vi "Welcome UI.vi"() -> ()   [LabVIEW 2016]
uses:
  <vilib>/Utility/error.llb/DialogType.ctl
  Architecture/Queue Management/ARC_Queue Create_Single.vi
  Architecture/Queue Management/ARC_Queue Valid.vi
  Architecture/Queue Management/ARC_Queue Insert Element.vi
  Architecture/Queue Management/ARC_Queue Remove Element.vi
  Architecture/Queue Management/ARC_Queue Destroy_Single.vi
panel:
  out "Logo":picture
  out "Title":string
  out "version":string
  in  "Parameter":cluster{"Q-Local":string, "Variant":variant}
  out "Error Report":string
  out "Current State":string
  in  "Exit Program":bool
  # "/* -------- Notes for All Users -------- */\nRecommand : \n[1].Display Setting Resolution -> 1440x900\n[2].Read Arch Notes First.\n[3].Make A Call When You Are In Trouble.\n\nTeam Members:\nPansino Soft,Pansino SDMA\n\nCopyright@2013 Pansino.Beijing\n\nVersion Number: 2013"
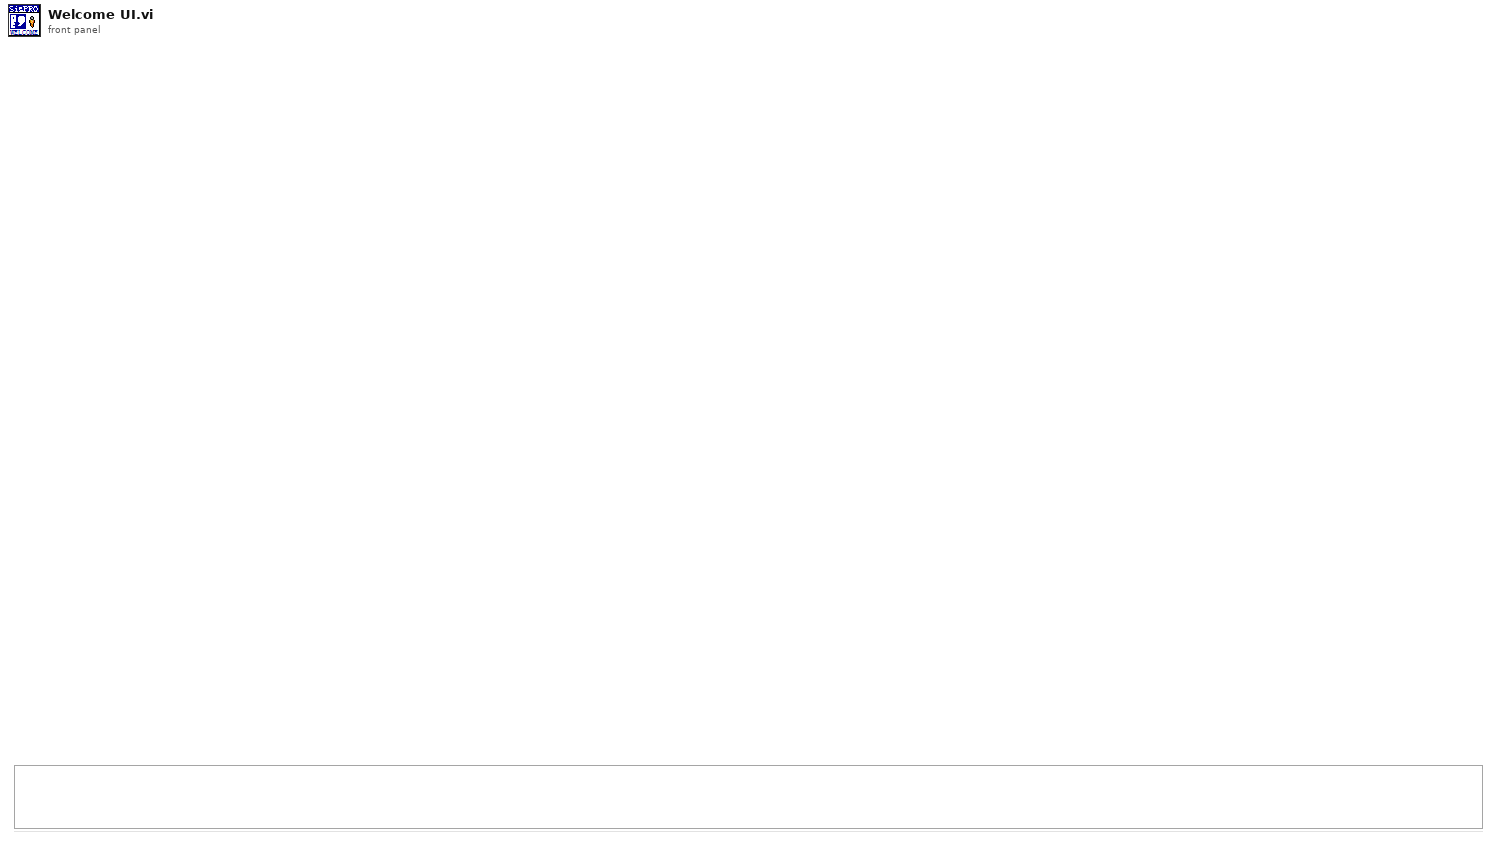
[diagram p1: front panel]
types:
  T1 = cluster{"Error":errorcluster, "Exit":bool, "System Path":cluster{"SysINI":path}, "Ref":cluster{"VIRef":refnum<vi>}, "Queue":cluster{"Q-Local":cluster{"Q-Local Name":string, "Q-Local Order":string, "Q-Local Data":variant}, "Q-HighLevel":cluster{"Q-HighLevel Name":string, "Q-HighLevel Order":string, "Q-HighLevel Data":variant}, "Q-LowLevel":cluster{"Q-LowLevel Name":string, "Q-LowLevel Order":string, "Q-LowLevel Data":variant}}}
  T2 = cluster{"LocalName":string, "System Config":path}
  T3 = typedef "DialogType.ctl" = u16
  T4 = cluster{"title":string, "version":string, "logo":path, "background":path}
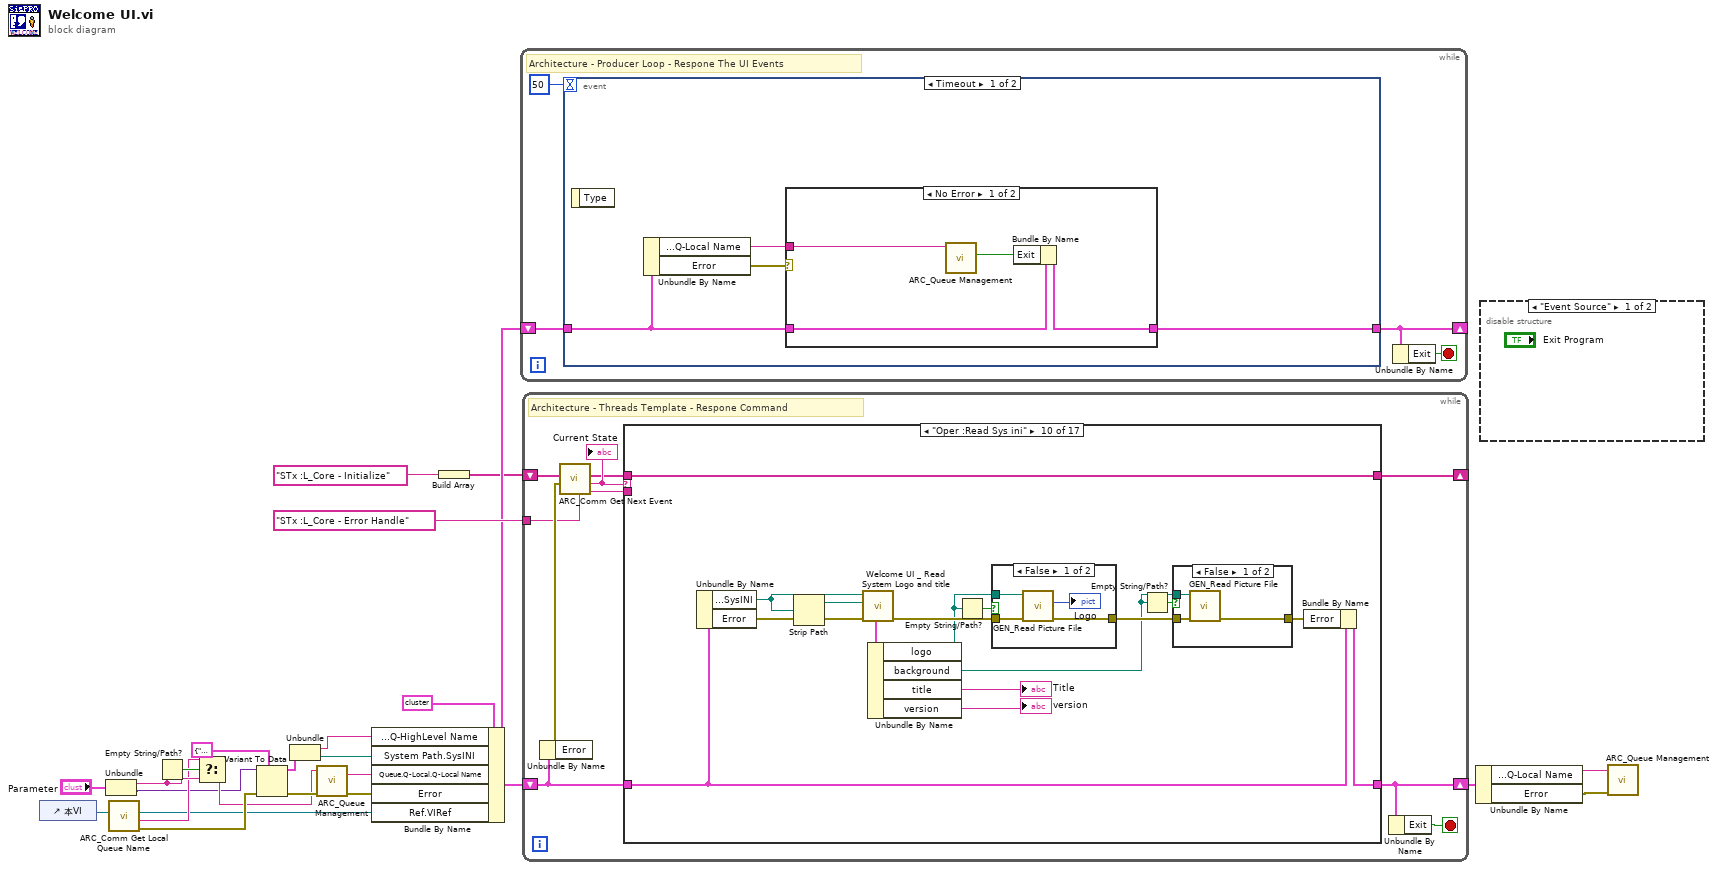
[diagram p0: block diagram]
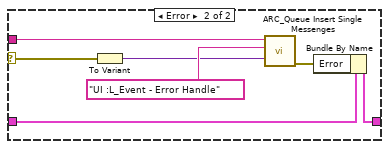
[diagram p2: hidden frame]
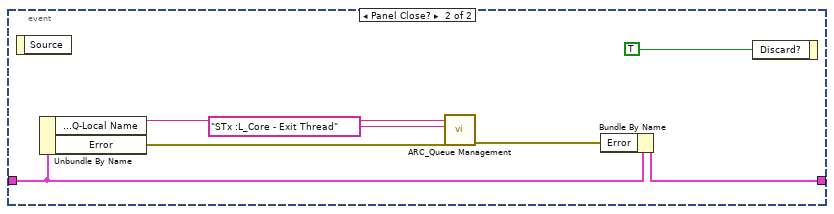
[diagram p3: hidden frame]
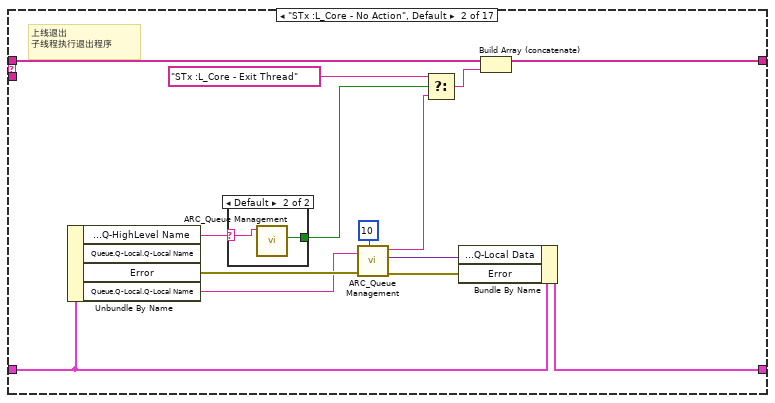
[diagram p6: hidden frame]
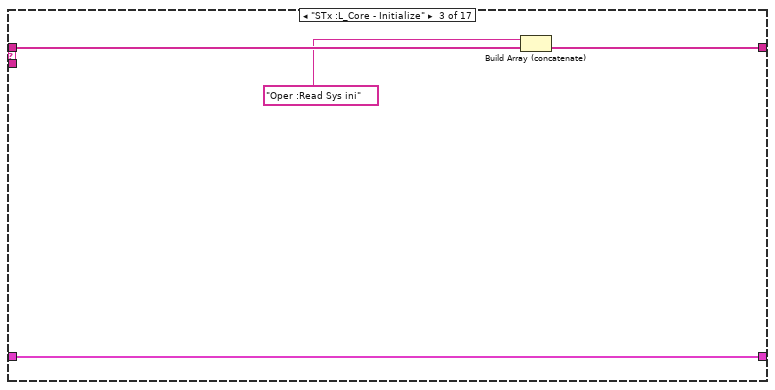
[diagram p8: hidden frame]
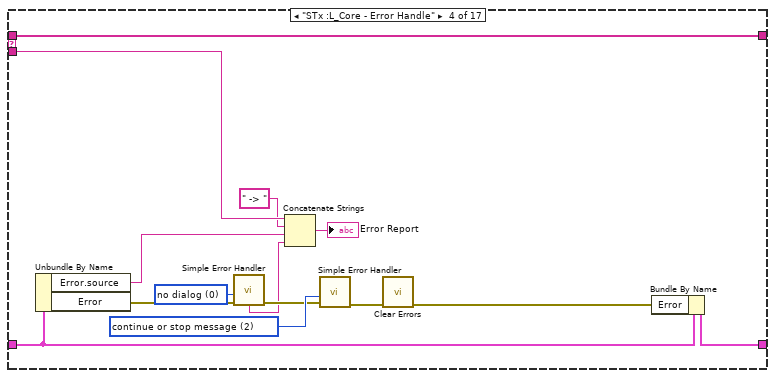
[diagram p9: hidden frame]
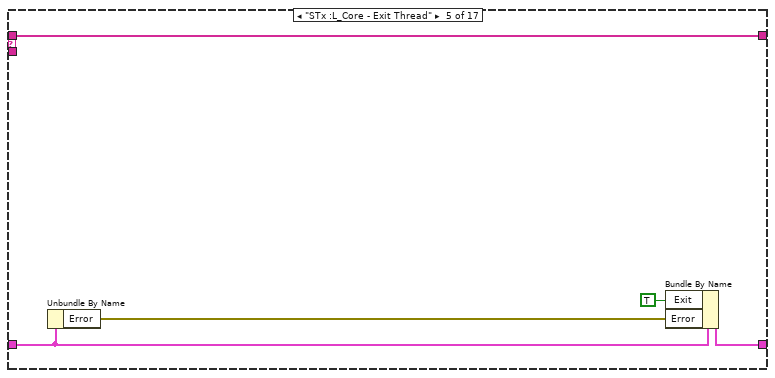
[diagram p10: hidden frame]
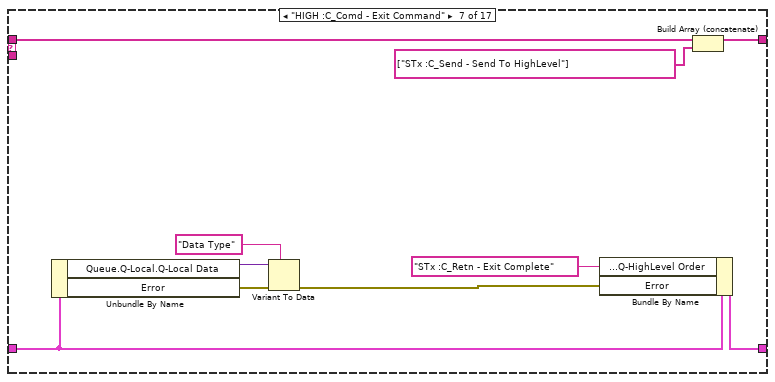
[diagram p12: hidden frame]
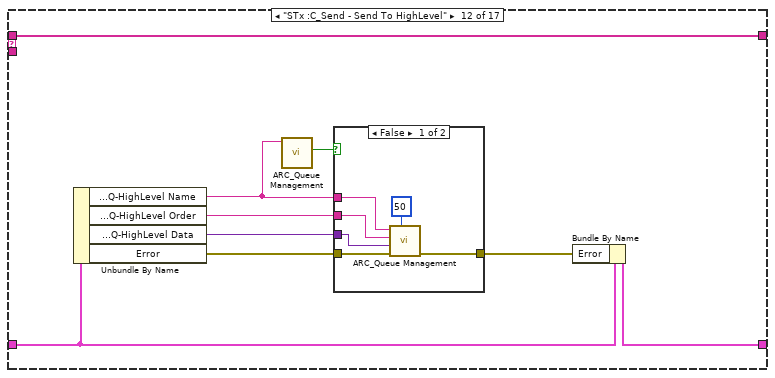
[diagram p18: hidden frame]
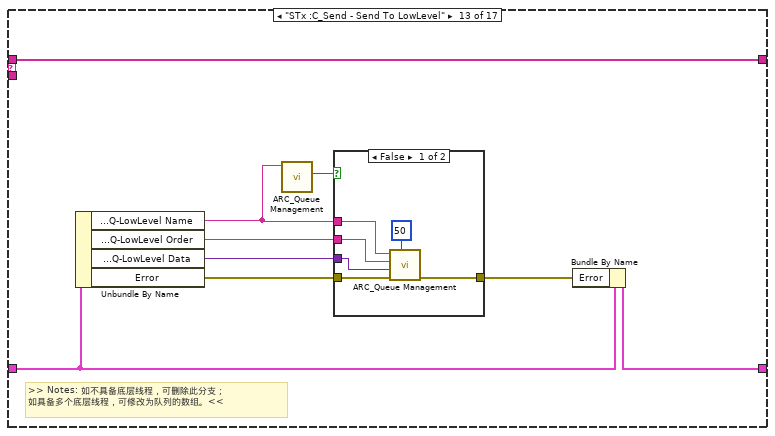
[diagram p20: hidden frame]
diagram:
  n1 = control-ref of="本VI"() -> (w13:refnum<vi>)
  n2 = Unbundle("Parameter") -> ("Q-Local"=w11:string, "Variant"=w6:variant)
  n3 = call "ARC_Comm Get Local Queue Name.vi"("VI Ref"=w13) -> ("error out"=w12:errorcluster, "VI  Name"=w9:string, "VI Ref out"=w5:refnum<vi>)  [unwired: 8 in]
  n4 = Empty String/Path?(string/path=w11) -> (empty?=w10:bool)
  n5 = Select(t=w9, s=w10, f=w11) -> (s? t:f=w8:string)
  n6 = Variant To Data(error in=w12, type=T2 {"LocalName"="", "System Config"=path ""} ("输出簇"), Variant=w6) -> (data=w3:T2, error out=w15:errorcluster)
  n7 = Unbundle(w3) -> ("LocalName"=w1:string, "System Config"=w2:path)
  n8 = call-poly "ARC_Queue Management.vi"("error in"=w15, "Queue Name"=w8) -> ("error out"=w24:errorcluster, "Queue Name dup"=w14:string)  [unwired: 7 in, 1 out]
  n9 = Bundle By Name(cluster=T1 {"Error"={"status"=FALSE, "code"=0, "source"=""}, "Exit"=FALSE, "System Path"={"SysINI"=path ""}, "Ref"={"VIRef"=refnum}, "Queue"={"Q-Local"={"Q-Local Name"="", "Q-Local Order"="", "Q-Local Data"=variant}, "Q-HighLevel"={"Q-HighLevel Name"="", "Q-HighLevel Order"="", "Q-HighLevel Data"=variant}, "Q-LowLevel"={"Q-LowLevel Name"="", "Q-LowLevel Order"="", "Q-LowLevel Data"=variant}}} ("TempVariable"), "Queue.Q-HighLevel.Q-HighLevel Name"=w1, "System Path.SysINI"=w2, "Queue.Q-Local.Q-Local Name"=w14, "Error"=w24, "Ref.VIRef"=w5) -> (w18:T1)
  n10 = Build Array("STx :L_Core - Initialize") -> (w16:string[])
  n11 = while {
    shift-right: [w26] -> _
    shift-left: w18 -> [w27]
    stop <- w25 stop-if-true
    # "Architecture - Producer Loop - Respone The UI Events"
    n12 = event shown="[0] Timeout" {
      selector: _ -> [_ _]
      dyn-events: _ -> [_ _]
      timeout: 50 -> [_ _]
      tunnel: w27 -> [w31 w48]
      tunnel: [w32 w47] -> w26
      event Timeout {
        n13 = event-data() -> ()  [unwired: 1 in, 1 out]
        n14 = Unbundle By Name(w31) -> ("Queue.Q-Local.Q-Local Name"=w30:string, "Error"=w29:errorcluster)
        n15 = case shown="No Error" w29 {
          selector: w29 -> [_ w43]
          tunnel: [w36 w41] -> w32
          tunnel: w31 -> [w34 w42]
          tunnel: w30 -> [w33 w40]
          frame No Error {
            n16 = call-poly "ARC_Queue Management.vi"("Queue Name(unamed)"=w33) -> ("Not Exist?"=w35:bool)  [unwired: 8 in, 2 out]
            n17 = Bundle By Name(cluster=w34, "Exit"=w35) -> (w36:T1)
          }
          frame Error {
            n18 = To Variant(anything=w43) -> (Variant=w38:variant)
            n19 = call "ARC_Queue Insert Single Messenges.vi"("Data"=w38, "Order"="UI :L_Event - Error Handle" ("Event"), "Queue Name"=w40) -> ("error out"=w37:errorcluster)  [unwired: 8 in]
            n20 = Bundle By Name(cluster=w42, "Error"=w37) -> (w41:T1)
          }
        }
      }
      event Panel Close? {
        n21 = event-data() -> ()  [unwired: 1 in, 1 out]
        n22 = Unbundle By Name(w48) -> ("Queue.Q-Local.Q-Local Name"=w45:string, "Error"=w49:errorcluster)
        n23 = call-poly "ARC_Queue Management.vi"("error in (no error)"=w49, "Event"="STx :L_Core - Exit Thread", "Queue Name(unamed)"=w45) -> ("error out"=w46:errorcluster)  [unwired: 7 in, 1 out]
        n24 = Bundle By Name(cluster=w48, "Error"=w46) -> (w47:T1)
        n25 = event-data("Discard?"=TRUE ("放弃？")) -> ()  [unwired: 1 in, 1 out]
      }
    }
    n26 = Unbundle By Name(w26) -> ("Exit"=w25:bool)
  }
  n27 = while {
    shift-right: [w54] -> w23
    shift-left: w18 -> [w56]
    shift-right: [w57] -> _
    shift-left: w16 -> [w60]
    tunnel: "STx :L_Core - Error Handle" ("Error Handle") -> [w52]
    stop <- w53 stop-if-true
    # "Architecture - Threads Template - Respone Command"
    n28 = Unbundle By Name(w56) -> ("Error"=w55:errorcluster)
    n29 = call "ARC_Comm Get Next Event.vi"("Error Handle"=w52, "error in (no error)"=w55, "event queue in"=w60) -> ("prev event"=w51:string, "next event"=w59:string, "event queue out"=w58:string[])  [unwired: 3 in]
    "Current State" <- w59
    n30 = case shown="\"Oper :Read Sys ini\"" w59 {
      tunnel: w56 -> [w61 w76 w79 w94 w98 w102 w110 w114 w116 w132 w143 w150 w166 w177 w182 w189 w195]
      tunnel: w58 -> [w62 w69 w82 w96 w101 w103 w113 w115 w117 w133 w144 w153 w169 w178 w180 w190 w193]
      tunnel: [w62 w68 w81 w96 w101 w103 w111 w115 w117 w133 w144 w153 w169 w178 w179 w190 w192] -> w57
      tunnel: [w61 w75 w79 w95 w99 w102 w112 w114 w116 w130 w143 w149 w165 w177 w181 w188 w194] -> w54
      tunnel: w51 -> [_ _ _ w87 _ _ _ _ _ _ _ _ _ _ _ _ _]
      frame "----------Core Status----------" {
      }
      frame "STx :L_Core - No Action", Default {
        # "上线退出\n子线程执行退出程序"
        n31 = Unbundle By Name(w76) -> ("Queue.Q-HighLevel.Q-HighLevel Name"=w71:string, "Error"=w72:errorcluster, "Queue.Q-Local.Q-Local Name"=w70:string)  [unwired: 1 out]
        n32 = case shown="Default" w71 {
          selector: w71 -> [_ w77]
          tunnel: [_ w78] -> w66
          frame "" {
          }
          frame Default {
            n33 = call-poly "ARC_Queue Management.vi"("Queue Name(unamed)"=w77) -> ("Not Exist?"=w78:bool)  [unwired: 8 in, 2 out]
          }
        }
        n34 = call-poly "ARC_Queue Management.vi"("Time out(-1)_queue out"=10, "error in (no error)"=w72, "Queue Name(unamed)"=w70) -> ("error out"=w74:errorcluster, "Data"=w73:variant, "Event"=w64:string)  [unwired: 5 in, 1 out]
        n35 = Select(t="STx :L_Core - Exit Thread" ("Event"), s=w66, f=w64) -> (s? t:f=w63:string)
        n36 = Bundle By Name(cluster=w76, "Queue.Q-Local.Q-Local Data"=w73, "Error"=w74) -> (w75:T1)
        n37 = Build Array (concatenate)(w69, w63) -> (w68:string[])
      }
      frame "STx :L_Core - Initialize" {
        n38 = Build Array (concatenate)("Oper :Read Sys ini", w82) -> (w81:string[])
      }
      frame "STx :L_Core - Error Handle" {
        w88 = T3 0 items=["no dialog", "OK message", "continue or stop message", "OK message + warnings", "continue/stop + warnings"] ("type of dialog (OK msg:1)")
        w91 = T3 2 items=["no dialog", "OK message", "continue or stop message", "OK message + warnings", "continue/stop + warnings"] ("type of dialog (OK msg:1)")
        n39 = Unbundle By Name(w94) -> ("Error.source"=w83:string, "Error"=w90:errorcluster)
        n40 = call <vilib>:"Simple Error Handler.vi"("type of dialog (OK msg:1)"=w88, "error in (no error)"=w90) -> ("error out"=w89:errorcluster, "message"=w85:string)  [unwired: 3 in, 3 out]
        n41 = Concatenate Strings(w87, " -> " ("字符串"), w83, w85) -> (→"Error Report":string)
        n42 = call <vilib>:"Simple Error Handler.vi"("type of dialog (OK msg:1)"=w91, "error in (no error)"=w89) -> ("error out"=w93:errorcluster)  [unwired: 3 in, 4 out]
        n43 = call <vilib>:"Clear Errors.vi"("error in (no error)"=w93) -> ("error out"=w92:errorcluster)  [unwired: 5 in, 1 out]
        n44 = Bundle By Name(cluster=w94, "Error"=w92) -> (w95:T1)
      }
      frame "STx :L_Core - Exit Thread" {
        n45 = Unbundle By Name(w98) -> ("Error"=w100:errorcluster)
        n46 = Bundle By Name(cluster=w98, "Exit"=TRUE, "Error"=w100) -> (w99:T1)
      }
      frame "----------Commond From HIGH----------" {
      }
      frame "HIGH :C_Comd - Exit Command" {
        n47 = Unbundle By Name(w110) -> ("Queue.Q-Local.Q-Local Data"=w109:variant, "Error"=w108:errorcluster)
        n48 = Variant To Data(error in=w108, type="Data Type" ("Data Type"), Variant=w109) -> (error out=w106:errorcluster)  [unwired: 1 out]
        n49 = Bundle By Name(cluster=w110, "Queue.Q-HighLevel.Q-HighLevel Order"="STx :C_Retn - Exit Complete" ("Data Type"), "Error"=w106) -> (w112:T1)
        n50 = Build Array (concatenate)(w113, string[] ["STx :C_Send - Send To HighLevel"] ("数组")) -> (w111:string[])
      }
      frame "----------Actions----------" {
      }
      frame "----------Operation----------" {
      }
      frame "Oper :Read Sys ini" {
        n51 = Unbundle By Name(w132) -> ("System Path.SysINI"=w120:path, "Error"=w131:errorcluster)
        n52 = Strip Path(path=w120) -> (stripped path=w119:path)  [unwired: 1 out]
        n53 = call "Welcome UI _ Read System Logo and title.vi"("error in"=w131, "file folder in"=w119, "file in"=w120) -> ("error out"=w129:errorcluster, "para out"=w127:T4)  [unwired: 7 in]
        n54 = Unbundle By Name(w127) -> ("logo"=w123:path, "background"=w125:path, "title"=→"Title":string, "version"=→"version":string)
        n55 = Empty String/Path?(string/path=w123) -> (empty?=w122:bool)
        n56 = case shown="False" w122 {
          tunnel: w129 -> [w137 w138]
          tunnel: [w136 w138] -> w128
          tunnel: w123 -> [w135 _]
          frame False {
            n57 = call "GEN_Read Picture File.vi"("error in"=w137, "file in"=w135) -> ("error out"=w136:errorcluster, "pic out"=→"Logo":picture)  [unwired: 8 in]
          }
          frame True {
          }
        }
        n58 = Empty String/Path?(string/path=w125) -> (empty?=w124:bool)
        n59 = case shown="False" w124 {
          tunnel: w128 -> [w141 w142]
          tunnel: w125 -> [w140 _]
          tunnel: [w139 w142] -> w126
          frame False {
            n60 = call "GEN_Read Picture File.vi"("error in"=w141, "file in"=w140) -> ("error out"=w139:errorcluster)  [unwired: 8 in, 1 out]
          }
          frame True {
          }
        }
        n61 = Bundle By Name(cluster=w132, "Error"=w126) -> (w130:T1)
      }
      frame "----------Communication----------" {
      }
      frame "STx :C_Send - Send To HighLevel" {
        n62 = Unbundle By Name(w150) -> ("Queue.Q-HighLevel.Q-HighLevel Name"=w152:string, "Queue.Q-HighLevel.Q-HighLevel Order"=w147:string, "Queue.Q-HighLevel.Q-HighLevel Data"=w146:variant, "Error"=w151:errorcluster)
        n63 = call-poly "ARC_Queue Management.vi"("Queue Name(unamed)"=w152) -> ("Not Exist?"=w148:bool)  [unwired: 8 in, 2 out]
        n64 = case shown="False" w148 {
          tunnel: w151 -> [w159 w160]
          tunnel: w152 -> [w157 _]
          tunnel: w147 -> [w155 _]
          tunnel: w146 -> [w156 _]
          tunnel: [w154 w160] -> w145
          frame False {
            n65 = call-poly "ARC_Queue Management.vi"("Time out(-1)_queue in"=50, "error in (no error)"=w159, "Data"=w156, "Event"=w155, "Queue Name(unamed)"=w157) -> ("error out"=w154:errorcluster)  [unwired: 5 in, 1 out]
          }
          frame True {
          }
        }
        n66 = Bundle By Name(cluster=w150, "Error"=w145) -> (w149:T1)
      }
      frame "STx :C_Send - Send To LowLevel" {
        # ">> Notes: 如不具备底层线程，可删除此分支；\n如具备多个底层线程，可修改为队列的数组。<<"
        n67 = Unbundle By Name(w166) -> ("Queue.Q-LowLevel.Q-LowLevel Name"=w168:string, "Queue.Q-LowLevel.Q-LowLevel Order"=w163:string, "Queue.Q-LowLevel.Q-LowLevel Data"=w162:variant, "Error"=w167:errorcluster)
        n68 = call-poly "ARC_Queue Management.vi"("Queue Name(unamed)"=w168) -> ("Not Exist?"=w164:bool)  [unwired: 8 in, 2 out]
        n69 = case shown="False" w164 {
          tunnel: w167 -> [w175 w176]
          tunnel: w168 -> [w173 _]
          tunnel: w163 -> [w171 _]
          tunnel: w162 -> [w172 _]
          tunnel: [w170 w176] -> w161
          frame False {
            n70 = call-poly "ARC_Queue Management.vi"("Time out(-1)_queue in"=50, "error in (no error)"=w175, "Data"=w172, "Event"=w171, "Queue Name(unamed)"=w173) -> ("error out"=w170:errorcluster)  [unwired: 5 in, 1 out]
          }
          frame True {
          }
        }
        n71 = Bundle By Name(cluster=w166, "Error"=w161) -> (w165:T1)
      }
      frame "----------Respond From LOW----------" {
      }
      frame "LOW :C_Resp - /* ADD NAME */" {
        n72 = Unbundle By Name(w182) -> ("Error"=w183:errorcluster)
        n73 = Build Array (concatenate)(w180) -> (w179:string[])
        n74 = Bundle By Name(cluster=w182, "Error"=w183) -> (w181:T1)
      }
      frame "LOW :C_Resp - /*Respond The Request*/" {
        n75 = Unbundle By Name(w189) -> ("Queue.Q-Local.Q-Local Data"=w186:variant, "Error"=w187:errorcluster)
        n76 = Variant To Data(error in=w187, type="Data Type" ("Data Type"), Variant=w186) -> (error out=w185:errorcluster)  [unwired: 1 out]
        n77 = Bundle By Name(cluster=w189, "Error"=w185) -> (w188:T1)
      }
      frame "LOW :C_Resp - Exit Complete" {
        # ">> Notes: 此处接收下层的返回指令；: 前代表下层的VI功能名，如ACTS等<<"
        n78 = Unbundle By Name(w195) -> ("Error"=w196:errorcluster)
        n79 = Build Array (concatenate)(w193, string[] ["STx :L_Core - Exit Thread"] ("数组")) -> (w192:string[])
        n80 = Bundle By Name(cluster=w195, "Error"=w196) -> (w194:T1)
      }
    }
    n81 = Unbundle By Name(w54) -> ("Exit"=w53:bool)
  }
  n82 = Unbundle By Name(w23) -> ("Queue.Q-Local.Q-Local Name"=w21:string, "Error"=w22:errorcluster)
  n83 = disable-structure shown="\"Event Source\"" {
    frame condition #0 (active) {
    }
    frame condition #1 {
    }
  }
  n84 = call-poly "ARC_Queue Management.vi"("error in (no error)"=w22, "Queue Name(unamed)"=w21) -> ()  [unwired: 7 in, 3 out]
